vi "Change ComboBox Strings.vi"(5 "index":i32, 6 "error in":errorcluster, 7 "Parameters":string[](array[string]), 8 "Control Name":string, 9 "VI reference in":refnum<vi>) -> (0 "error out":errorcluster, 3 "VI reference out":refnum<vi>)   [LabVIEW 2020, in "Scheduler.lvlib"]
doc: "VI for updating the string combobox with list of parameters. VI gets a reference to the SubPanel VI, Name of the Control with the ComboBox, Index of the element in a cluster containing ComboBox, and list of parameters to in the ComboBox"
uses:
  Scheduler.lvlib
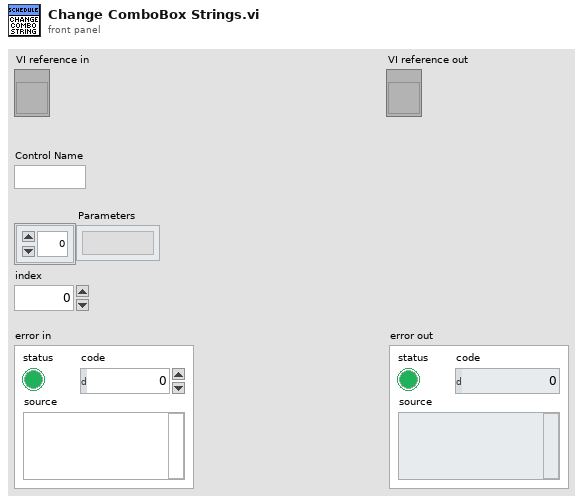
[diagram p1: front panel]
types:
  T1 = cluster{"Parameter Name":string, "Parameter Name":string}
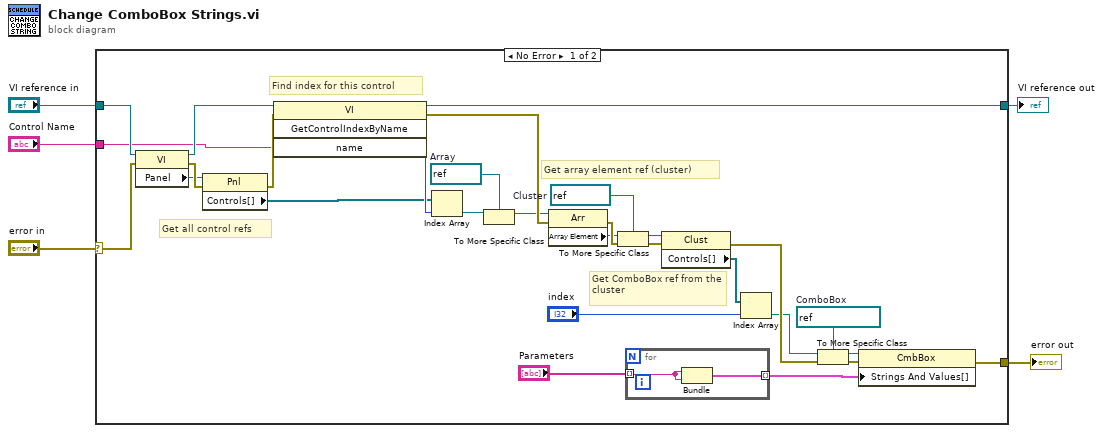
[diagram p0: block diagram]
diagram:
  n1 = case shown="No Error" "error in" {
    selector: "error in" -> [w11 w38]
    tunnel: [w25 w38] -> w5
    tunnel: "Control Name" -> [w7 _]
    tunnel: "VI reference in" -> [w12 w37]
    tunnel: [w6 w37] -> w1
    frame No Error {
      w17 = refnum<vi> refnum  # Cluster
      w18 = refnum<vi> refnum  # Array
      w28 = refnum<vi> refnum  # ComboBox
      # "Get array element ref (cluster)"
      # "Get ComboBox ref from the cluster"
      # "Find index for this control"
      # "Get all control refs"
      n2 = property class="VI"(reference=w12, error in=w11) -> (reference out=w10:refnum<vi>, error out=w14:errorcluster, "Panel"=w13:refnum<vi>)
      n3 = property class="Pnl"(reference=w13, error in=w14) -> (error out=w9:errorcluster, "Controls[]"=w8:refnum<vi>[])  [unwired: 1 out]
      n4 = invoke class="VI" method="GetControlIndexByName"(reference=w10, error in=w9, "name"=w7) -> (reference out=w6:refnum<vi>, error out=w32:errorcluster, "GetControlIndexByName"=w21:i32)  [unwired: 1 in, 1 out]
      n5 = Index Array(array=w8, index=w21) -> (element=w20:refnum<vi>)
      n6 = To More Specific Class(target class=w18, reference=w20) -> (specific class reference=w19:refnum<vi>)  [unwired: 1 in, 1 out]
      n7 = property class="Arr"(reference=w19, error in=w32) -> (error out=w33:errorcluster, "Array Element"=w22:refnum<vi>)  [unwired: 1 out]
      n8 = To More Specific Class(target class=w17, reference=w22, error in=w33) -> (specific class reference=w23:refnum<vi>, error out=w15:errorcluster)
      n9 = for {
        tunnel: "Parameters" -> [w36] mode=indexing
        tunnel: [w35] -> w27 mode=indexing
        n10 = Bundle("Parameter Name"=w36, "Parameter Name"=w36) -> (w35:T1)  [unwired: 1 in]
      }
      n11 = property class="Clust"(reference=w23, error in=w15) -> (error out=w34:errorcluster, "Controls[]"=w16:refnum<vi>[])  [unwired: 1 out]
      n12 = Index Array(array=w16, index="index") -> (element=w29:refnum<vi>)
      n13 = To More Specific Class(target class=w28, reference=w29, error in=w34) -> (specific class reference=w31:refnum<vi>, error out=w30:errorcluster)
      n14 = property class="CmbBox"(reference=w31, error in=w30, "Strings And Values[]"=w27) -> (error out=w25:errorcluster)  [unwired: 1 out]
    }
    frame Error {
    }
  }
  "error out" <- w5
  "VI reference out" <- w1
